vi "Search for existing item.vi"(10 "Line":T2, 11 "Array":T5[](array[typedef])) -> (0 "New Quantity":u32, 1 "Found Quantity":u32, 2 "Found?":bool, 3 "Output Arrays":T1)   [LabVIEW 2013]
uses:
  Controls/Display Component Line.ctl
  Controls/Components.ctl
  Controls/Component Sub Type.ctl
  Controls/Add Button.ctl
  Controls/Subtract Button.ctl
  Controls/Add Component Line.ctl
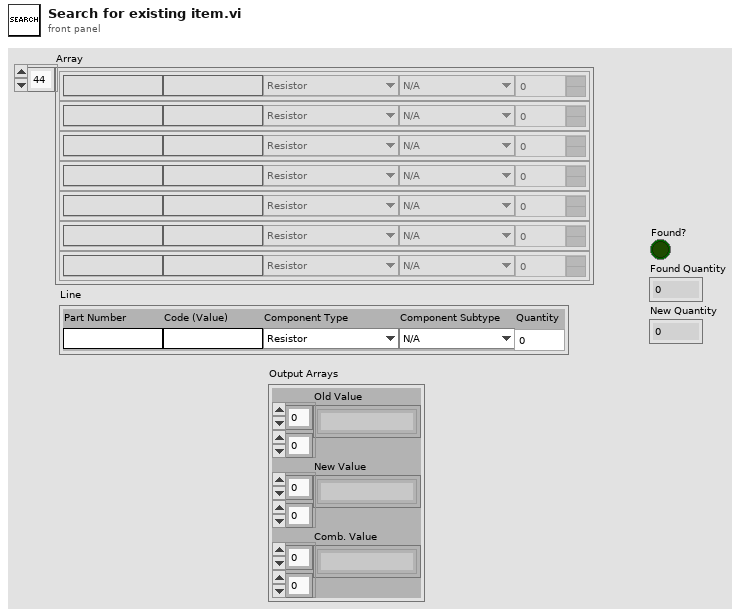
[diagram p1: front panel]
types:
  T1 = cluster{"Old Value":string[][], "New Value":string[][], "Comb. Value":string[][]}
  T2 = typedef "Add Component Line.ctl" = cluster{"Part Number":string, "Code (Value)":string, "Component Type":T3, "Component Subtype":T4, "Quantity":u32}
  T3 = typedef "Components.ctl" = enum16{"Resistor", "Capacitor", "Diode", "Voltage Regulator", "Transistors", "ICs", "Misc"}
  T4 = typedef "Component Sub Type.ctl" = enum16{"N/A", "Carbon", "Variable - Trimmer", "Variable - Pot", "Ceramic", "Electrolitic", "Zenner", "TO-92", "TO-220", "NPN", "PNP", "CMOS", "Processor"}
  T5 = typedef "Display Component Line.ctl" = cluster{"Part Number":string, "Code (Value)":string, "Component Type":T3, "Component Subtype":T4, "Quantity":u32, "Add":T6, "Subtract":T7}
  T6 = typedef "Add Button.ctl" = bool
  T7 = typedef "Subtract Button.ctl" = bool
  T8 = cluster{"Part Number":bool, "Code (Value)":bool, "Component Type":bool, "Component Subtype":bool, "Quantity":bool, "Add":T6, "Subtract":T7}
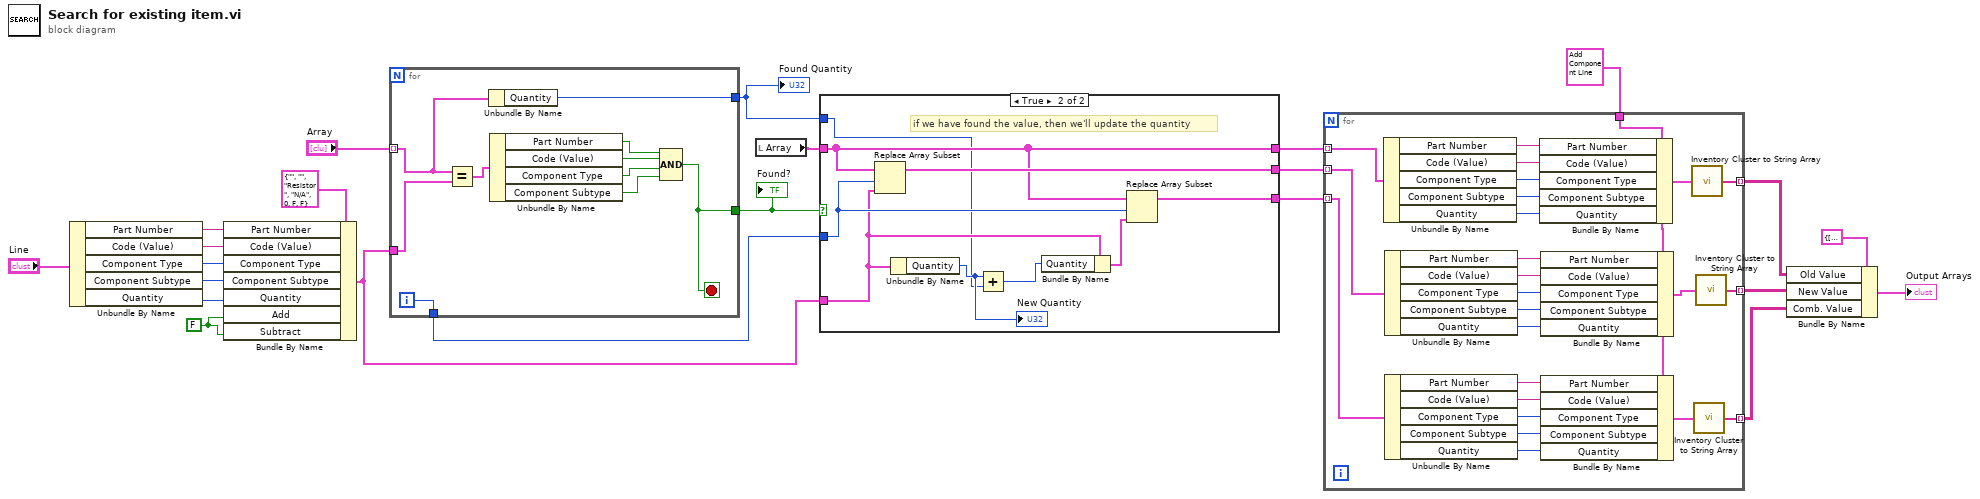
[diagram p0: block diagram]
diagram:
  w15 = FALSE
  n1 = Unbundle By Name("Line") -> ("Part Number"=w20:string, "Code (Value)"=w19:string, "Component Type"=w18:T3, "Component Subtype"=w17:T4, "Quantity"=w16:u32)
  n2 = Bundle By Name(cluster=T5 {"Part Number"="", "Code (Value)"="", "Component Type"=enum."Resistor", "Component Subtype"=enum."N/A", "Quantity"=0, "Add"=FALSE, "Subtract"=FALSE} ("Display Components Line"), "Part Number"=w20, "Code (Value)"=w19, "Component Type"=w18, "Component Subtype"=w17, "Quantity"=w16, "Add"=w15, "Subtract"=w15) -> (w12:T5)
  n3 = for {
    tunnel: "Array" -> [w25] mode=indexing
    tunnel: w12 -> [w33]
    tunnel: [w27] -> w13
    tunnel: [w26] -> w14
    tunnel: [w24] -> w10
    i -> [w27]
    stop <- w26 stop-if-true
    n4 = Equal?(x=w25, y=w33) -> (x = y?=w32:T8)
    n5 = Unbundle By Name(w25) -> ("Quantity"=w24:u32)
    n6 = Unbundle By Name(w32) -> ("Part Number"=w31:bool, "Code (Value)"=w30:bool, "Component Type"=w29:bool, "Component Subtype"=w28:bool)
    n7 = Compound Arithmetic op=AND(w31, w30, w29, w28) -> (w26:bool)
  }
  "Found?" <- w14
  "Found Quantity" <- w10
  n8 = local read "Array"() -> (w11:T5[])
  n9 = case shown="True" w14 {
    tunnel: w13 -> [_ w41]
    tunnel: w12 -> [_ w40]
    tunnel: [w34 w43] -> w8
    tunnel: [w34 w42] -> w9
    tunnel: w11 -> [w34 w42]
    tunnel: w10 -> [_ w38]
    tunnel: [w34 w35] -> w7
    frame False {
    }
    frame True {
      # "if we have found the value, then we'll update the quantity"
      n10 = Replace Array Subset(array=w42, new element=w40, index=w41) -> (w43:T5[])
      n11 = Unbundle By Name(w40) -> ("Quantity"=w39:u32)
      "New Quantity" <- w39
      n12 = Add(x=w39, y=w38) -> (x+y=w37:u32)
      n13 = Bundle By Name(cluster=w40, "Quantity"=w37) -> (w36:T5)
      n14 = Replace Array Subset(array=w42, new element=w36, index=w41) -> (w35:T5[])
    }
  }
  n15 = for {
    tunnel: w9 -> [w68] mode=indexing
    tunnel: w8 -> [w49] mode=indexing
    tunnel: w7 -> [w48] mode=indexing
    tunnel: T2 {"Part Number"="", "Code (Value)"="10M", "Component Type"=enum."Resistor", "Component Subtype"=enum."Carbon", "Quantity"=50} ("Component Line") -> [w50]
    tunnel: [w61] -> w3 mode=indexing
    tunnel: [w45] -> w2 mode=indexing
    tunnel: [w44] -> w4 mode=indexing
    n16 = Unbundle By Name(w68) -> ("Part Number"=w67:string, "Code (Value)"=w66:string, "Component Type"=w65:T3, "Component Subtype"=w64:T4, "Quantity"=w63:u32)
    n17 = Unbundle By Name(w49) -> ("Part Number"=w56:string, "Code (Value)"=w57:string, "Component Type"=w58:T3, "Component Subtype"=w59:T4, "Quantity"=w60:u32)
    n18 = Unbundle By Name(w48) -> ("Part Number"=w55:string, "Code (Value)"=w54:string, "Component Type"=w53:T3, "Component Subtype"=w52:T4, "Quantity"=w51:u32)
    n19 = Bundle By Name(cluster=w50, "Part Number"=w67, "Code (Value)"=w66, "Component Type"=w65, "Component Subtype"=w64, "Quantity"=w63) -> (w62:T2)
    n20 = Bundle By Name(cluster=w50, "Part Number"=w56, "Code (Value)"=w57, "Component Type"=w58, "Component Subtype"=w59, "Quantity"=w60) -> (w46:T2)
    n21 = Bundle By Name(cluster=w50, "Part Number"=w55, "Code (Value)"=w54, "Component Type"=w53, "Component Subtype"=w52, "Quantity"=w51) -> (w47:T2)
    n22 = call "Inventory Cluster to String Array.vi"("Component Line"=w62) -> ("Array"=w61:string[])
    n23 = call "Inventory Cluster to String Array.vi"("Component Line"=w47) -> ("Array"=w44:string[])
    n24 = call "Inventory Cluster to String Array.vi"("Component Line"=w46) -> ("Array"=w45:string[])
  }
  n25 = Bundle By Name(cluster=T1 {"Old Value"=[], "New Value"=[], "Comb. Value"=[]} ("Output Arrays"), "Old Value"=w3, "New Value"=w2, "Comb. Value"=w4) -> (→"Output Arrays":T1)
